vi "object-generation-speedtest.vi"(8 "error in (no error)":errorcluster) -> (0 "error out":errorcluster)   [LabVIEW 2013]
uses:
  src/SMO/SMO.lvclass
  <vilib>/addons/_JKI Toolkits/Caraya/classes/Test/Test.lvclass
  <vilib>/addons/_JKI Toolkits/Caraya/classes/Assert/Assert.lvclass
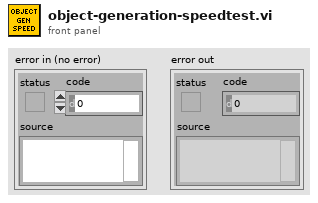
[diagram p1: front panel]
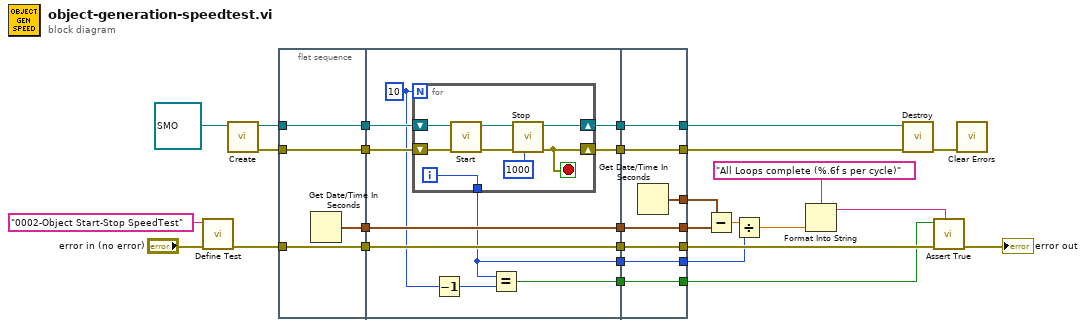
[diagram p0: block diagram]
diagram:
  n1 = call <vilib>:"Define Test.vi"("error in (no error)"="error in (no error)", "Label (VI Title)"="0002-Object Start-Stop SpeedTest") -> ("error out"=w20:errorcluster)  [unwired: 9 in]
  n2 = call "Create.vi"("SMO"=refnum<class "SMO.lvclass"> refnum ("SMO.lvclass")) -> ("error out"=w24:errorcluster, "SMO out"=w25:refnum<class "SMO.lvclass">)  [unwired: 8 in, 1 out]
  n3 = flat-sequence {
    tunnel: w20 -> [w31]
    tunnel: w24 -> [w32]
    tunnel: w25 -> [w33]
    tunnel: [w33] -> w15
    tunnel: [w32] -> w14
    tunnel: [w31] -> w13
    tunnel: [w30] -> w11
    tunnel: [w41] -> w18
    tunnel: [w40] -> w17
    tunnel: [w39] -> w16
    tunnel: w15 -> [w43]
    tunnel: w14 -> [w42]
    tunnel: w13 -> [w39]
    tunnel: [w38] -> w12
    tunnel: w11 -> [w38]
    tunnel: [w37] -> w8
    tunnel: [w34] -> w4
    tunnel: [w56] -> w19
    tunnel: [w57] -> w22
    tunnel: [w58] -> w23
    tunnel: w18 -> [w58]
    tunnel: w17 -> [w57]
    tunnel: w16 -> [w56]
    tunnel: [w55] -> w10
    tunnel: w12 -> [w55]
    tunnel: [w54] -> w9
    tunnel: [w53] -> w6
    tunnel: w8 -> [w53]
    tunnel: [w52] -> w5
    tunnel: w4 -> [w52]
    frame #0 {
      n4 = Get Date/Time In Seconds() -> (seconds since 1Jan1904=w30:timestamp)
    }
    frame #1 {
      w36 = 10
      n5 = for {
        N: w36 -> [_]
        shift-right: [w47] -> w41
        shift-left: w43 -> [w51]
        shift-right: [w45] -> w40
        shift-left: w42 -> [w50]
        tunnel: [w44] -> w37
        i -> [w44]
        stop <- w45 stop-if-true
        n6 = call "Start.vi"("error in (no error)"=w50, "SMO"=w51) -> ("error out"=w48:errorcluster, "SMO out"=w49:refnum<class "SMO.lvclass">)  [unwired: 8 in]
        n7 = call "Stop.vi"("timeout in ms (-1)"=1000, "error in (no error)"=w48, "SMO"=w49) -> ("error out"=w45:errorcluster, "SMO out"=w47:refnum<class "SMO.lvclass">)  [unwired: 7 in]
      }
      n8 = Decrement(x=w36) -> (x-1=w35:i32)
      n9 = Equal?(x=w37, y=w35) -> (x = y?=w34:bool)
    }
    frame #2 {
      n10 = Get Date/Time In Seconds() -> (seconds since 1Jan1904=w54:timestamp)
    }
  }
  n11 = Subtract(x=w9, y=w10) -> (x-y=w7:dbl)
  n12 = Divide(x=w7, y=w6) -> (x/y=w3:dbl)
  n13 = Format Into String(format string="All Loops complete (%.6f s per cycle)" ("Label (VI Title)"), w3) -> (resulting string=w1:string)  [unwired: 2 in, 1 out]
  n14 = call "Destroy.vi"("error in (no error)"=w22, "SMO"=w23) -> ("error out"=w21:errorcluster)  [unwired: 9 in]
  n15 = call <vilib>:"Assert True.vi"("Label"=w1, "error in (no error)"=w19, "True?"=w5) -> ("error out"=→"error out":errorcluster)  [unwired: 8 in]
  n16 = call <vilib>:"Clear Errors.vi"("error in (no error)"=w21) -> ()  [unwired: 6 in, 1 out]
